vi "Create render window_3Dpf.vi"(0 "Camera Controller:Type":T1(ring)=enum."Oriented", 2 "Up Direction":T2={"X"=0.0, "Y"=0.0, "Z"=1.0}, 3 "Scene in":refnum<vi>, 4 "Target":T2, 5 "Camera Position":T2={"X"=3000.0, "Y"=0.0, "Z"=1000.0}, 6 "Height":i16=1080, 7 "Width":i16=1920) -> (1 "Scene out":refnum<vi>)   [LabVIEW 2017]
doc: "Creates a render window of specified size and camera control mode for a given scene."
uses:
  <vilib>/Utility/miscctls.llb/LV3DPointTypeDef.ctl
  <vilib>/Utility/miscctls.llb/LVRectTypeDef.ctl
  <vilib>/picture/3D Picture Control/NI_3D Picture Control.lvlib
panel:
  # "PN 03/02/2015"
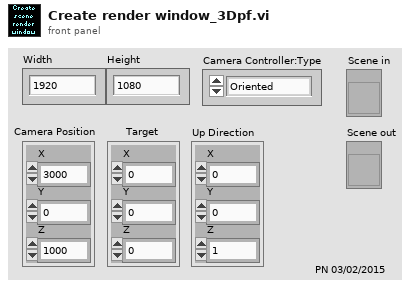
[diagram p1: front panel]
types:
  T1 = enum16{"None", "Spherical", "Flying", "Oriented"}
  T2 = typedef "LV3DPointTypeDef.ctl" = cluster{"X":sgl, "Y":sgl, "Z":sgl}
  T3 = typedef "LVRectTypeDef.ctl" = cluster{"Left":i16, "Top":i16, "Right":i16, "Bottom":i16}
  T4 = enum16{"Open", "Minimized", "Maximized", "Hidden"}
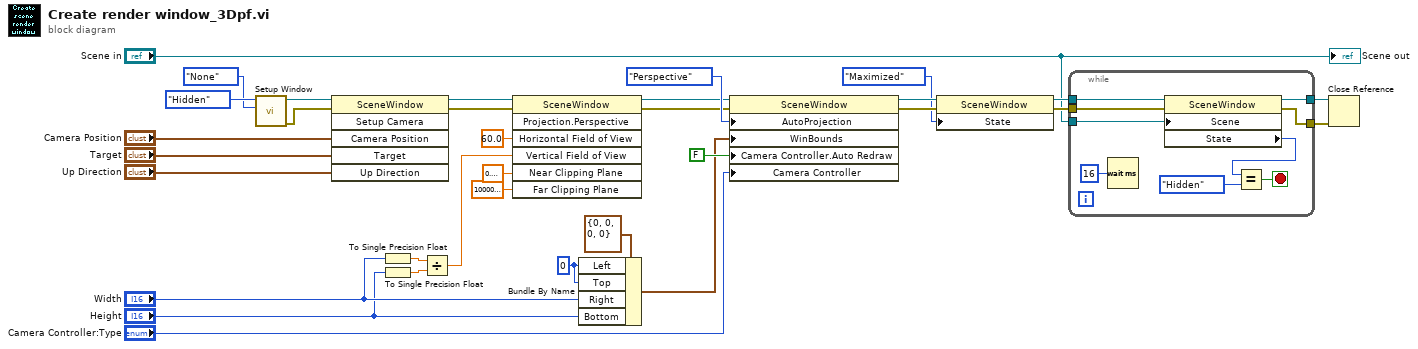
[diagram p0: block diagram]
diagram:
  w9 = i16 0 ("Left")
  n1 = call <vilib>:"Setup Window.vi"("Camera Controller"=enum16{"None", "Spherical", "Flying"}."None", "Window State"=T4."Hidden") -> ("error out"=w27:errorcluster, "New Window Refnum"=w28:refnum<vi>)  [unwired: 8 in]
  n2 = invoke class="SceneWindow" method="Setup Camera"(reference=w28, error in=w27, "Camera Position"="Camera Position", "Target"="Target", "Up Direction"="Up Direction") -> (reference out=w12:refnum<vi>, error out=w14:errorcluster)  [unwired: 1 in, 4 out]
  n3 = To Single Precision Float(number="Width") -> (single precision float=w7:sgl)
  n4 = To Single Precision Float(number="Height") -> (single precision float=w6:sgl)
  n5 = Divide(x=w7, y=w6) -> (x/y=w3:sgl)
  n6 = invoke class="SceneWindow" method="Projection.Perspective"(reference=w12, error in=w14, "Horizontal Field of View"=sgl 60.0 ("Field of View"), "Vertical Field of View"=w3, "Near Clipping Plane"=sgl 0.1, "Far Clipping Plane"=sgl 1000000.0) -> (reference out=w11:refnum<vi>, error out=w13:errorcluster)  [unwired: 1 in, 5 out]
  n7 = Bundle By Name(cluster=T3 {"Left"=0, "Top"=0, "Right"=0, "Bottom"=0} ("Window Bounds"), "Left"=w9, "Top"=w9, "Right"="Width", "Bottom"="Height") -> (w8:T3)
  n8 = property class="SceneWindow"(reference=w11, error in=w13, "AutoProjection"=enum16{"None", "Perspective", "Orthographic"}."Perspective" ("Automatic Projection Mode"), "WinBounds"=w8, "Camera Controller.Auto Redraw"=FALSE ("Camera Controller:Auto Redraw"), "Camera Controller"="Camera Controller:Type") -> (reference out=w24:refnum<vi>, error out=w23:errorcluster)
  n9 = property class="SceneWindow"(reference=w24, error in=w23, "State"=T4."Maximized" ("Window State")) -> (reference out=w21:refnum<vi>, error out=w20:errorcluster)
  n10 = while {
    tunnel: w21 -> [w38]
    tunnel: w20 -> [w42]
    tunnel: [w35] -> w19
    tunnel: [w41] -> w18
    tunnel: "Scene in" -> [w34]
    stop <- w39 stop-if-true
    n11 = Wait (ms)(milliseconds to wait=u32 16) -> ()  [unwired: 1 out]
    n12 = property class="SceneWindow"(reference=w38, error in=w42, "Scene"=w34) -> (reference out=w35:refnum<vi>, error out=w41:errorcluster, "State"=w36:T4)
    n13 = Equal?(x=w36, y=T4."Hidden" ("Window State")) -> (x = y?=w39:bool)
  }
  n14 = Close Reference(reference=w19, error in (no error)=w18) -> ()  [unwired: 1 out]
  "Scene out" <- "Scene in"
